vi "Time Data Filtering (V1.00).vi"(0 "wFormDSP ref in":refnum<class "GSwFormDSP.lvclass">, 5 "error in (no error)":errorcluster, 7 "Application Name":string="GenUtil", 9 "State Queue":string[](array[string])=["SC >>> Initialize"]) -> (19 "error out":errorcluster)   [LabVIEW 2022 SP3, in "SigMath.lvclass"]
uses:
  SigMath.lvclass
  API/GSwFormDSP_class/GSwFormDSP.lvclass
  <vilib>/Analysis/2dsp.llb/1D Convolution (DBL).vi
  <vilib>/Analysis/2dsp.llb/Complex FFT.vi
  W:/projects/archives/23 Charette AI Group/SPWB/API/Generic Utilities_class/Generic Utilities.lvclass
  <vilib>/Analysis/baseanly.llb/IIR Cascade Filter (DBL).vi
  API/Generic Utilities_class/Generic Utilities.lvclass
  <vilib>/Analysis/NI_AALBase.lvlib
  <vilib>/Analysis/NI_AALPro.lvlib
  <vilib>/addons/_AddQ/G#Object/G#Object.lvclass
  File IO/TDMS_class/TDMS.lvclass
panel:
  in  "GUI View":enum32{"Interface", "Admin"}(tab)
  in  "Filter Source":T1(ring)
  out "Magnitude Graph":dbl[](graph)
  out "Phase Graph":dbl[](graph)
  out "Fs":dbl
  in  "Phaseless Filter":bool=TRUE
  in  "passband ripple (dB)":dbl=0.1 caption="Passband\nRipple (dB)" format="%.2f"
  in  "stopband attenuation (dB)":dbl=60.0 caption="Stopband\nAttenuation (dB)" format="%.2f"
  in  "Order":i32=8
  in  "Type":T2(ring)=enum."Elliptic"
  in  "Upper Cut Off Freq":dbl=1000.0 format="%#.3f"
  in  "Cut Off Freq":dbl=600.0 format="%#.3f"
  in  "Filter":T3(ring)
  in  "Include Fade IN and OUT":bool
  in  "Apply":bool
  out "State History":string[](array[string])
  out "State Index":i32
  # "Filter Response"
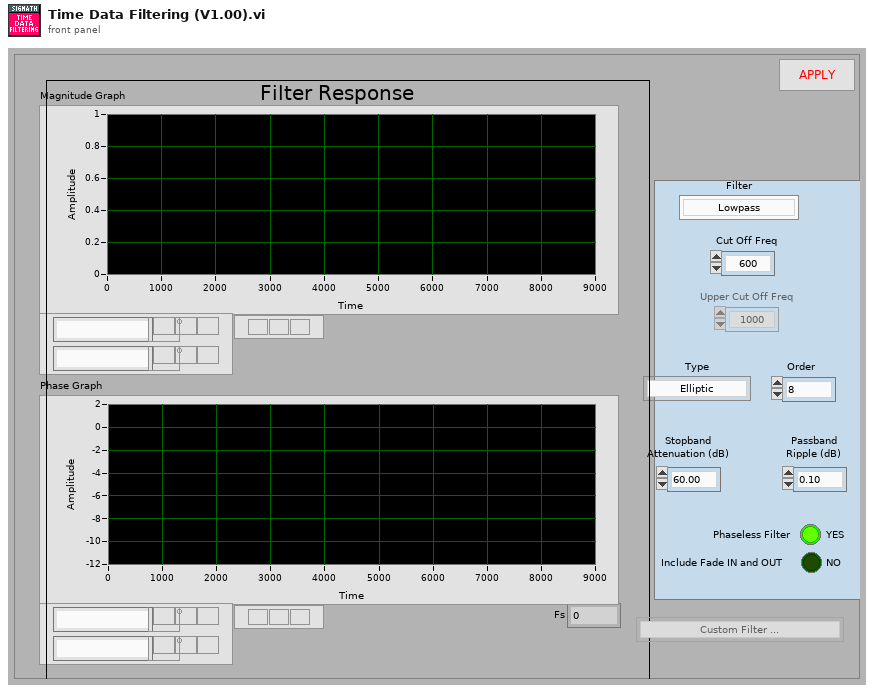
[diagram p1: front panel]
types:
  T1 = enum16{"Custom Filter ...", "Import Impulse Response (TDMS File)"}
  T2 = enum16{"Butterworth", "Chebyshev", "Inv Chebyshev", "Elliptic", "Bessel"}
  T3 = enum32{"Lowpass", "Highpass", "Bandpass", "Bandstop"}
  T4 = enum32{"Invalid", "Standard", "Closed", "Hidden", "Minimized", "Maximized"}
  T5 = enum8{"Enabled", "Disabled", "Disabled and Grayed Out"}
  T6 = typedef "SigMath.lvclass/SigMath Data.ctl" = cluster{"New Time Data Obj?":bool, "GSwFormDSP":refnum<class "GSwFormDSP.lvclass">}
  T7 = typedef "GSwFormDSP.lvclass/TDF Parameters.ctl" = cluster{"Filter":enum32{"Lowpass", "Highpass", "Bandpass", "Bandstop"}, "Type:":enum16{"Butterworth", "Chebyshev", "Inv Chebyshev", "Elliptic", "Bessel"}, "LP cutoff freq":dbl, "HP cutoff freq":dbl, "Order":i32, "passband ripple (dB)":dbl, "stopband attenuation (dB)":dbl, "Phaseless Filter":bool, "Include Fade IN and OUT":bool}
  T8 = cluster{"filter structure":enum32{"IIR 2nd Order", "IIR 4th Order"}, "Reverse Coefficients":dbl[], "Forward Coefficients":dbl[]}
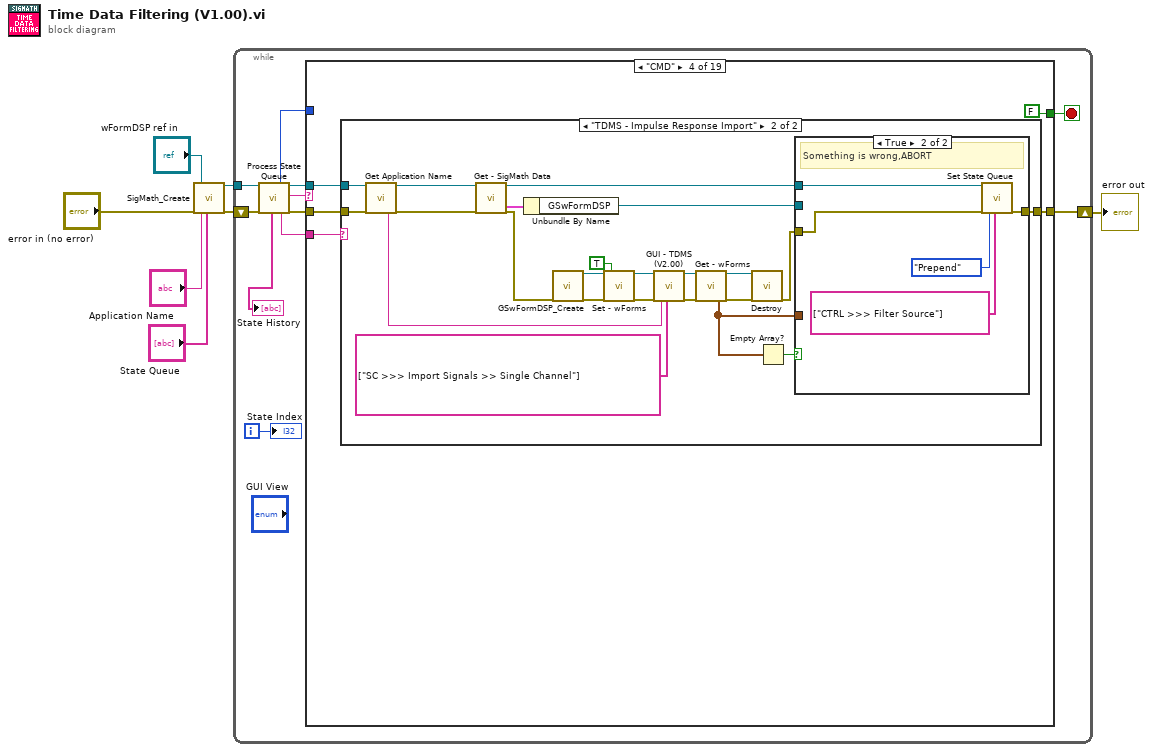
[diagram p0: block diagram]
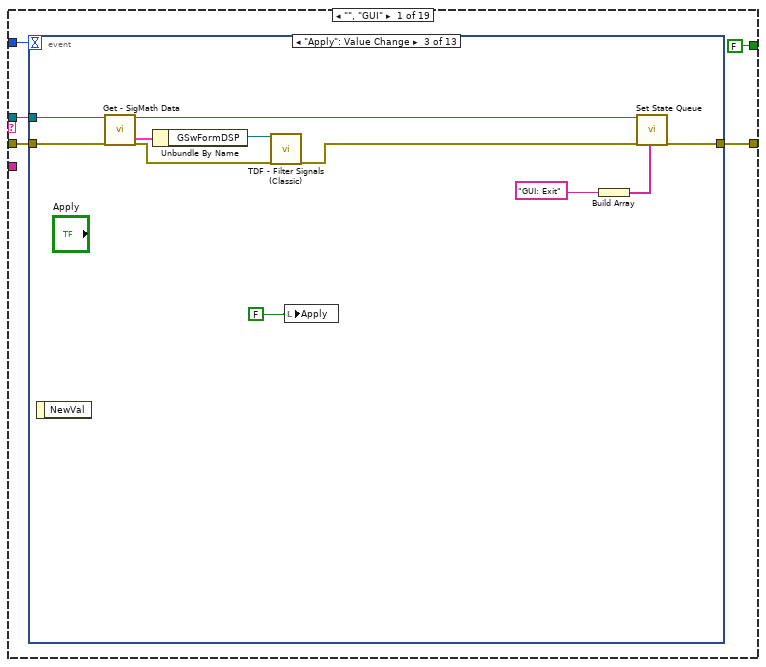
[diagram p2: hidden frame]
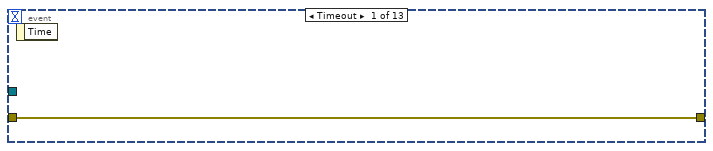
[diagram p3: hidden frame]
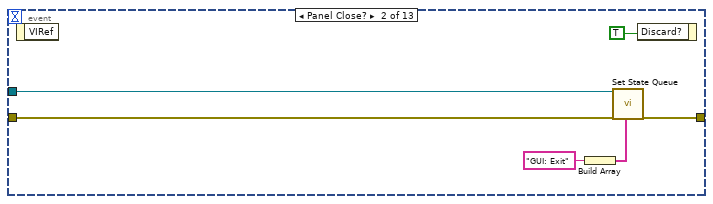
[diagram p4: hidden frame]
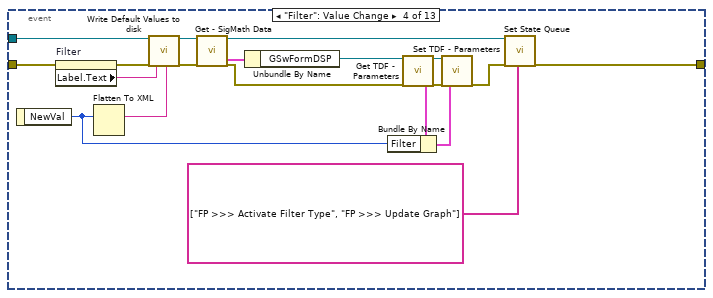
[diagram p5: hidden frame]
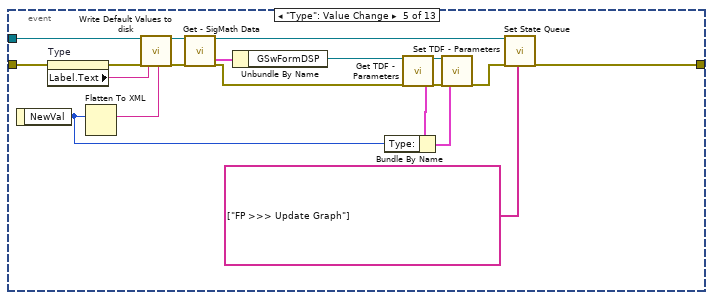
[diagram p6: hidden frame]
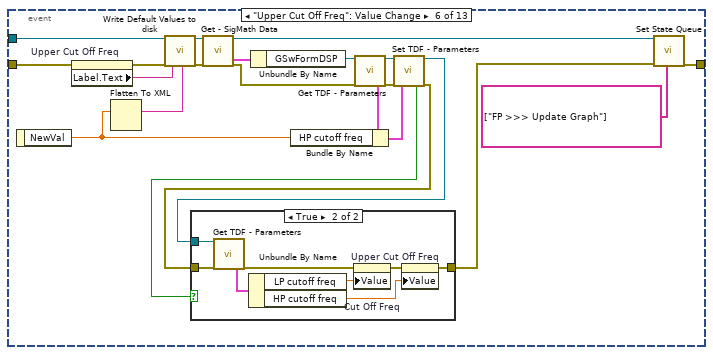
[diagram p7: hidden frame]
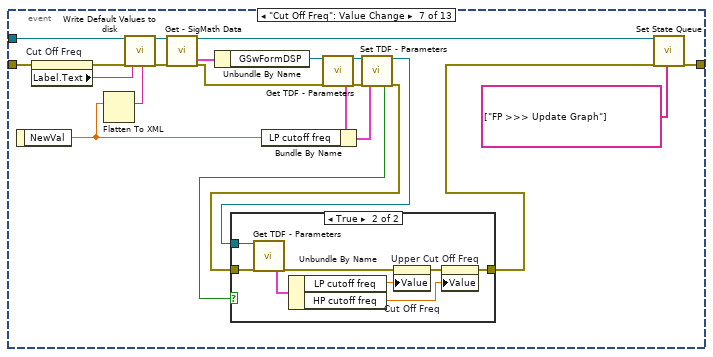
[diagram p9: hidden frame]
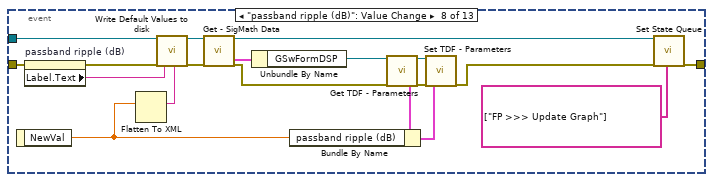
[diagram p11: hidden frame]
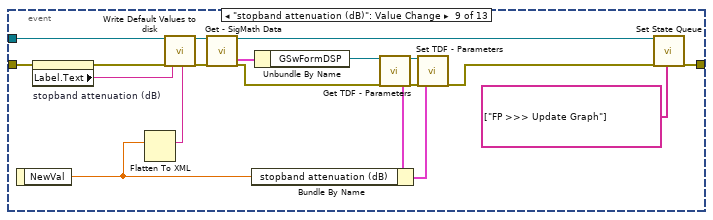
[diagram p12: hidden frame]
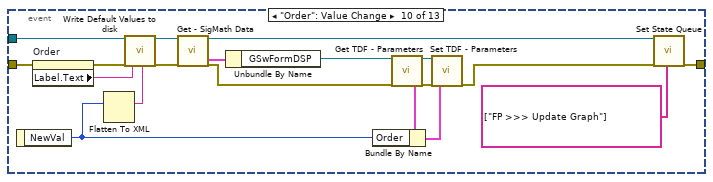
[diagram p13: hidden frame]
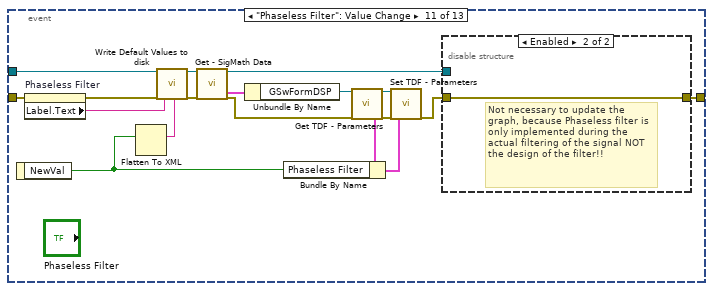
[diagram p14: hidden frame]
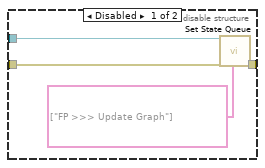
[diagram p15: hidden frame]
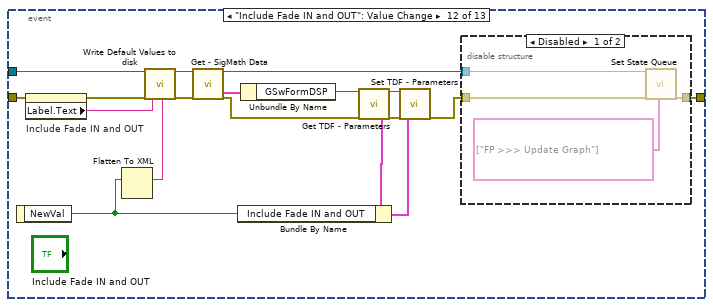
[diagram p16: hidden frame]
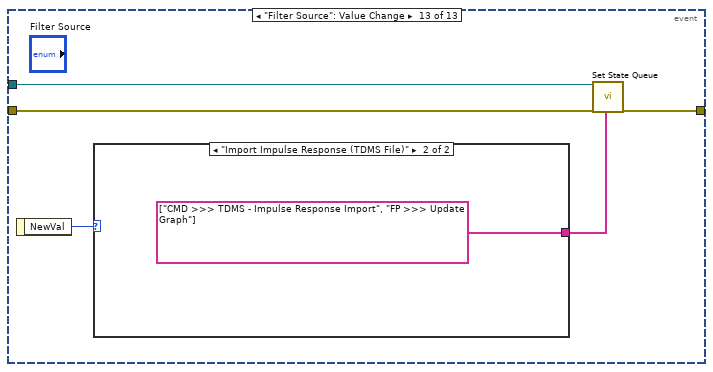
[diagram p18: hidden frame]
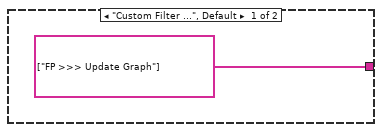
[diagram p19: hidden frame]
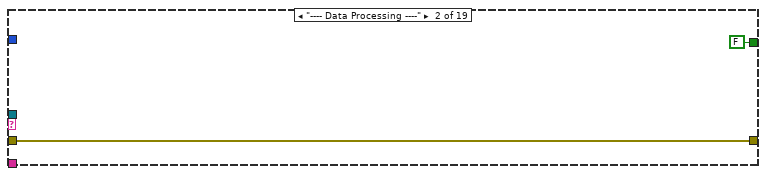
[diagram p20: hidden frame]
diagram:
  n1 = call "SigMath_Create.vi"("error in (no error)"="error in (no error)", "Time Data"="wFormDSP ref in", "Application Name"="Application Name", "State Queue"="State Queue") -> ("reference out"=w7:refnum<class "SigMath.lvclass">, "error out"=w6:errorcluster)  [unwired: 14 in]
  n2 = while {
    shift-right: [w10] -> w2
    shift-left: w6 -> [w15]
    tunnel: w7 -> [w16]
    i -> [w17]
    stop <- w18 stop-if-true
    n3 = call "Process State Queue.vi"("reference in"=w16, "error in (no error)"=w15) -> ("State History"=→"State History":string[], "Timeout"=w14:i32, "State Option"=w9:string, "reference out"=w13:refnum<class "SigMath.lvclass">, "Current State"=w12:string, "error out"=w11:errorcluster)  [unwired: 10 in, 2 out]
    n4 = case shown="\"CMD\"" w12 {
      selector: w12 -> [_ _ _ _ _ _ _ _ _ _ _ _ _ _ _ w812 _ _ _]
      tunnel: w13 -> [w21 _ _ w256 _ w306 _ w319 w609 _ w720 w733 w769 w794 _ _ _ _ w822]
      tunnel: [FALSE FALSE FALSE FALSE FALSE FALSE FALSE FALSE FALSE FALSE FALSE TRUE FALSE FALSE FALSE FALSE FALSE FALSE TRUE] -> w18
      tunnel: w14 -> [w22 _ _ _ _ _ _ _ _ _ _ _ _ _ _ _ _ _ _]
      tunnel: w9 -> [_ _ _ w259 _ w302 _ w320 w606 _ _ _ w778 _ _ _ _ _ _]
      tunnel: w11 -> [w20 w252 w254 w257 w299 w305 w315 w317 w608 w711 w716 w730 w768 w795 w808 w810 w815 w818 w821]
      tunnel: [w19 w252 w254 w258 w299 w304 w315 w318 w607 w711 w717 w729 w766 w791 w808 w810 errorcluster {"status"=FALSE, "code"=0, "source"=""} ("error out") w818 w820] -> w10
      frame "", "GUI" {
        n5 = event shown="[2] \"Apply\": Value Change" {
          selector: _ -> [_ _ _ _ _ _ _ _ _ _ _ _ _]
          dyn-events: _ -> [_ _ _ _ _ _ _ _ _ _ _ _ _]
          timeout: w22 -> [_ _ _ _ _ _ _ _ _ _ _ _ _]
          tunnel: w21 -> [_ w28 w36 w60 w79 w92 w123 w150 w169 w188 w207 w230 w246]
          tunnel: w20 -> [w24 w27 w35 w57 w76 w91 w122 w149 w168 w187 w206 w229 w247]
          tunnel: [w24 w26 w40 w48 w67 w93 w124 w151 w170 w189 w208 w231 w248] -> w19
          event Timeout {
            n6 = event-data() -> ()  [unwired: 1 in, 1 out]
          }
          event Panel Close? {
            n7 = event-data() -> ()  [unwired: 1 in, 1 out]
            n8 = Build Array("GUI: Exit") -> (w25:string[])
            n9 = call "Set State Queue.vi"("reference in"=w28, "error in (no error)"=w27, "State Queue"=w25) -> ("error out"=w26:errorcluster)  [unwired: 15 in, 1 out]
            n10 = event-data("Discard?"=TRUE) -> ()  [unwired: 1 in, 1 out]
          }
          event "Apply": Value Change {
            n11 = event-data() -> ()  [unwired: 1 in, 1 out]
            n12 = call "Get - SigMath Data.vi"("reference in"=w36, "error in (no error)"=w35) -> ("SigMath Data"=w37:T6, "reference out"=w31:refnum<class "SigMath.lvclass">, "error out"=w33:errorcluster)  [unwired: 15 in]
            n13 = Unbundle By Name(w37) -> ("GSwFormDSP"=w34:refnum<class "GSwFormDSP.lvclass">)
            n14 = call "TDF - Filter Signals (Classic).vi"("reference in"=w34, "error in (no error)"=w33) -> ("error out"=w32:errorcluster)  [unwired: 16 in, 1 out]
            n15 = local write "Apply"(FALSE ("Exit")) -> ()
            n16 = Build Array("GUI: Exit") -> (w39:string[])
            n17 = call "Set State Queue.vi"("reference in"=w31, "error in (no error)"=w32, "State Queue"=w39) -> ("error out"=w40:errorcluster)  [unwired: 15 in, 1 out]
          }
          event "Filter": Value Change {
            n18 = event-data() -> ("NewVal"=w54:T3)  [unwired: 1 in]
            n19 = property on="Filter" class="Enum (strict)"(error in=w57) -> (error out=w56:errorcluster, "Label.Text"=w59:string)  [unwired: 1 in, 1 out]
            n20 = Flatten To XML(6:w54) -> (2:w58:string)
            n21 = call-dynamic "Write Default Values to disk.vi"("reference in"=w60, "error in (no error)"=w56, "Control Label"=w59, "Value (XML String)"=w58) -> ("reference out"=w46:refnum<class "SigMath.lvclass">, "error out"=w45:errorcluster)  [unwired: 14 in]
            n22 = call "Get - SigMath Data.vi"("reference in"=w46, "error in (no error)"=w45) -> ("SigMath Data"=w47:T6, "reference out"=w43:refnum<class "SigMath.lvclass">, "error out"=w42:errorcluster)  [unwired: 15 in]
            n23 = Unbundle By Name(w47) -> ("GSwFormDSP"=w44:refnum<class "GSwFormDSP.lvclass">)
            n24 = call "Get TDF - Parameters.vi"("reference in"=w44, "error in (no error)"=w42) -> ("TDF Parameters"=w55:T7, "reference out"=w53:refnum<class "GSwFormDSP.lvclass">, "error out"=w52:errorcluster)  [unwired: 15 in]
            n25 = Bundle By Name(cluster=w55, "Filter"=w54) -> (w51:T7)
            n26 = call "Set TDF - Parameters.vi"("reference in"=w53, "error in (no error)"=w52, "TDF Parameters"=w51) -> ("error out"=w50:errorcluster)  [unwired: 14 in, 2 out]
            n27 = call "Set State Queue.vi"("reference in"=w43, "error in (no error)"=w50, "State Queue"=string[] ["FP >>> Activate Filter Type", "FP >>> Update Graph"]) -> ("error out"=w48:errorcluster)  [unwired: 15 in, 1 out]
          }
          event "Type": Value Change {
            n28 = event-data() -> ("NewVal"=w73:T2)  [unwired: 1 in]
            n29 = property on="Type" class="Enum (strict)"(error in=w76) -> (error out=w75:errorcluster, "Label.Text"=w78:string)  [unwired: 1 in, 1 out]
            n30 = Flatten To XML(6:w73) -> (2:w77:string)
            n31 = call-dynamic "Write Default Values to disk.vi"("reference in"=w79, "error in (no error)"=w75, "Control Label"=w78, "Value (XML String)"=w77) -> ("reference out"=w65:refnum<class "SigMath.lvclass">, "error out"=w64:errorcluster)  [unwired: 14 in]
            n32 = call "Get - SigMath Data.vi"("reference in"=w65, "error in (no error)"=w64) -> ("SigMath Data"=w66:T6, "reference out"=w61:refnum<class "SigMath.lvclass">, "error out"=w62:errorcluster)  [unwired: 15 in]
            n33 = Unbundle By Name(w66) -> ("GSwFormDSP"=w63:refnum<class "GSwFormDSP.lvclass">)
            n34 = call "Get TDF - Parameters.vi"("reference in"=w63, "error in (no error)"=w62) -> ("TDF Parameters"=w74:T7, "reference out"=w72:refnum<class "GSwFormDSP.lvclass">, "error out"=w71:errorcluster)  [unwired: 15 in]
            n35 = Bundle By Name(cluster=w74, "Type:"=w73) -> (w70:T7)
            n36 = call "Set TDF - Parameters.vi"("reference in"=w72, "error in (no error)"=w71, "TDF Parameters"=w70) -> ("error out"=w69:errorcluster)  [unwired: 14 in, 2 out]
            n37 = call "Set State Queue.vi"("reference in"=w61, "error in (no error)"=w69, "State Queue"=string[] ["FP >>> Update Graph"]) -> ("error out"=w67:errorcluster)  [unwired: 15 in, 1 out]
          }
          event "Upper Cut Off Freq": Value Change {
            n38 = event-data() -> ("NewVal"=w90:dbl)  [unwired: 1 in]
            n39 = property on="Upper Cut Off Freq" class="DigNum (strict)"(error in=w91) -> (error out=w99:errorcluster, "Label.Text"=w101:string)  [unwired: 1 in, 1 out]
            n40 = Flatten To XML(6:w90) -> (2:w100:string)
            n41 = call-dynamic "Write Default Values to disk.vi"("reference in"=w92, "error in (no error)"=w99, "Control Label"=w101, "Value (XML String)"=w100) -> ("reference out"=w84:refnum<class "SigMath.lvclass">, "error out"=w83:errorcluster)  [unwired: 14 in]
            n42 = call "Get - SigMath Data.vi"("reference in"=w84, "error in (no error)"=w83) -> ("SigMath Data"=w85:T6, "reference out"=w80:refnum<class "SigMath.lvclass">, "error out"=w82:errorcluster)  [unwired: 15 in]
            n43 = Unbundle By Name(w85) -> ("GSwFormDSP"=w81:refnum<class "GSwFormDSP.lvclass">)
            n44 = call "Get TDF - Parameters.vi"("reference in"=w81, "error in (no error)"=w82) -> ("TDF Parameters"=w98:T7, "reference out"=w97:refnum<class "GSwFormDSP.lvclass">, "error out"=w96:errorcluster)  [unwired: 15 in]
            n45 = Bundle By Name(cluster=w98, "HP cutoff freq"=w90) -> (w95:T7)
            n46 = call "Set TDF - Parameters.vi"("reference in"=w97, "error in (no error)"=w96, "TDF Parameters"=w95) -> ("Cut Off Freq. Coerced?"=w88:bool, "reference out"=w86:refnum<class "GSwFormDSP.lvclass">, "error out"=w89:errorcluster)  [unwired: 14 in]
            n47 = case shown="True" w88 {
              tunnel: [w102 w105] -> w87
              tunnel: w89 -> [w102 w110]
              tunnel: w86 -> [_ w109]
              frame False {
              }
              frame True {
                n48 = call "Get TDF - Parameters.vi"("reference in"=w109, "error in (no error)"=w110) -> ("TDF Parameters"=w108:T7, "error out"=w106:errorcluster)  [unwired: 15 in, 1 out]
                n49 = Unbundle By Name(w108) -> ("LP cutoff freq"=w107:dbl, "HP cutoff freq"=w103:dbl)
                n50 = property on="Cut Off Freq" class="DigNum (strict)"(error in=w106, "Value"=w107) -> (error out=w104:errorcluster)  [unwired: 1 in, 1 out]
                n51 = property on="Upper Cut Off Freq" class="DigNum (strict)"(error in=w104, "Value"=w103) -> (error out=w105:errorcluster)  [unwired: 1 in, 1 out]
              }
            }
            n52 = call "Set State Queue.vi"("reference in"=w80, "error in (no error)"=w87, "State Queue"=string[] ["FP >>> Update Graph"]) -> ("error out"=w93:errorcluster)  [unwired: 15 in, 1 out]
          }
          event "Cut Off Freq": Value Change {
            n53 = event-data() -> ("NewVal"=w121:dbl)  [unwired: 1 in]
            n54 = property on="Cut Off Freq" class="DigNum (strict)"(error in=w122) -> (error out=w130:errorcluster, "Label.Text"=w132:string)  [unwired: 1 in, 1 out]
            n55 = Flatten To XML(6:w121) -> (2:w131:string)
            n56 = call-dynamic "Write Default Values to disk.vi"("reference in"=w123, "error in (no error)"=w130, "Control Label"=w132, "Value (XML String)"=w131) -> ("reference out"=w115:refnum<class "SigMath.lvclass">, "error out"=w114:errorcluster)  [unwired: 14 in]
            n57 = call "Get - SigMath Data.vi"("reference in"=w115, "error in (no error)"=w114) -> ("SigMath Data"=w116:T6, "reference out"=w111:refnum<class "SigMath.lvclass">, "error out"=w112:errorcluster)  [unwired: 15 in]
            n58 = Unbundle By Name(w116) -> ("GSwFormDSP"=w113:refnum<class "GSwFormDSP.lvclass">)
            n59 = call "Get TDF - Parameters.vi"("reference in"=w113, "error in (no error)"=w112) -> ("TDF Parameters"=w129:T7, "reference out"=w128:refnum<class "GSwFormDSP.lvclass">, "error out"=w127:errorcluster)  [unwired: 15 in]
            n60 = Bundle By Name(cluster=w129, "LP cutoff freq"=w121) -> (w126:T7)
            n61 = call "Set TDF - Parameters.vi"("reference in"=w128, "error in (no error)"=w127, "TDF Parameters"=w126) -> ("Cut Off Freq. Coerced?"=w117:bool, "reference out"=w120:refnum<class "GSwFormDSP.lvclass">, "error out"=w119:errorcluster)  [unwired: 14 in]
            n62 = case shown="True" w117 {
              tunnel: [w133 w136] -> w118
              tunnel: w119 -> [w133 w141]
              tunnel: w120 -> [_ w140]
              frame False {
              }
              frame True {
                n63 = call "Get TDF - Parameters.vi"("reference in"=w140, "error in (no error)"=w141) -> ("TDF Parameters"=w139:T7, "error out"=w137:errorcluster)  [unwired: 15 in, 1 out]
                n64 = Unbundle By Name(w139) -> ("LP cutoff freq"=w138:dbl, "HP cutoff freq"=w134:dbl)
                n65 = property on="Cut Off Freq" class="DigNum (strict)"(error in=w137, "Value"=w138) -> (error out=w135:errorcluster)  [unwired: 1 in, 1 out]
                n66 = property on="Upper Cut Off Freq" class="DigNum (strict)"(error in=w135, "Value"=w134) -> (error out=w136:errorcluster)  [unwired: 1 in, 1 out]
              }
            }
            n67 = call "Set State Queue.vi"("reference in"=w111, "error in (no error)"=w118, "State Queue"=string[] ["FP >>> Update Graph"]) -> ("error out"=w124:errorcluster)  [unwired: 15 in, 1 out]
          }
          event "passband ripple (dB)": Value Change {
            n68 = event-data() -> ("NewVal"=w148:dbl)  [unwired: 1 in]
            n69 = property on="passband ripple (dB)" class="DigNum (strict)"(error in=w149) -> (error out=w158:errorcluster, "Label.Text"=w160:string)  [unwired: 1 in, 1 out]
            n70 = Flatten To XML(6:w148) -> (2:w159:string)
            n71 = call-dynamic "Write Default Values to disk.vi"("reference in"=w150, "error in (no error)"=w158, "Control Label"=w160, "Value (XML String)"=w159) -> ("reference out"=w146:refnum<class "SigMath.lvclass">, "error out"=w145:errorcluster)  [unwired: 14 in]
            n72 = call "Get - SigMath Data.vi"("reference in"=w146, "error in (no error)"=w145) -> ("SigMath Data"=w147:T6, "reference out"=w142:refnum<class "SigMath.lvclass">, "error out"=w143:errorcluster)  [unwired: 15 in]
            n73 = Unbundle By Name(w147) -> ("GSwFormDSP"=w144:refnum<class "GSwFormDSP.lvclass">)
            n74 = call "Get TDF - Parameters.vi"("reference in"=w144, "error in (no error)"=w143) -> ("TDF Parameters"=w157:T7, "reference out"=w156:refnum<class "GSwFormDSP.lvclass">, "error out"=w155:errorcluster)  [unwired: 15 in]
            n75 = Bundle By Name(cluster=w157, "passband ripple (dB)"=w148) -> (w154:T7)
            n76 = call "Set TDF - Parameters.vi"("reference in"=w156, "error in (no error)"=w155, "TDF Parameters"=w154) -> ("error out"=w153:errorcluster)  [unwired: 14 in, 2 out]
            n77 = call "Set State Queue.vi"("reference in"=w142, "error in (no error)"=w153, "State Queue"=string[] ["FP >>> Update Graph"]) -> ("error out"=w151:errorcluster)  [unwired: 15 in, 1 out]
          }
          event "stopband attenuation (dB)": Value Change {
            n78 = event-data() -> ("NewVal"=w167:dbl)  [unwired: 1 in]
            n79 = property on="stopband attenuation (dB)" class="DigNum (strict)"(error in=w168) -> (error out=w177:errorcluster, "Label.Text"=w179:string)  [unwired: 1 in, 1 out]
            n80 = Flatten To XML(6:w167) -> (2:w178:string)
            n81 = call-dynamic "Write Default Values to disk.vi"("reference in"=w169, "error in (no error)"=w177, "Control Label"=w179, "Value (XML String)"=w178) -> ("reference out"=w165:refnum<class "SigMath.lvclass">, "error out"=w164:errorcluster)  [unwired: 14 in]
            n82 = call "Get - SigMath Data.vi"("reference in"=w165, "error in (no error)"=w164) -> ("SigMath Data"=w166:T6, "reference out"=w162:refnum<class "SigMath.lvclass">, "error out"=w161:errorcluster)  [unwired: 15 in]
            n83 = Unbundle By Name(w166) -> ("GSwFormDSP"=w163:refnum<class "GSwFormDSP.lvclass">)
            n84 = call "Get TDF - Parameters.vi"("reference in"=w163, "error in (no error)"=w161) -> ("TDF Parameters"=w176:T7, "reference out"=w175:refnum<class "GSwFormDSP.lvclass">, "error out"=w174:errorcluster)  [unwired: 15 in]
            n85 = Bundle By Name(cluster=w176, "stopband attenuation (dB)"=w167) -> (w173:T7)
            n86 = call "Set TDF - Parameters.vi"("reference in"=w175, "error in (no error)"=w174, "TDF Parameters"=w173) -> ("error out"=w172:errorcluster)  [unwired: 14 in, 2 out]
            n87 = call "Set State Queue.vi"("reference in"=w162, "error in (no error)"=w172, "State Queue"=string[] ["FP >>> Update Graph"]) -> ("error out"=w170:errorcluster)  [unwired: 15 in, 1 out]
          }
          event "Order": Value Change {
            n88 = event-data() -> ("NewVal"=w186:i32)  [unwired: 1 in]
            n89 = property on="Order" class="DigNum (strict)"(error in=w187) -> (error out=w196:errorcluster, "Label.Text"=w198:string)  [unwired: 1 in, 1 out]
            n90 = Flatten To XML(6:w186) -> (2:w197:string)
            n91 = call-dynamic "Write Default Values to disk.vi"("reference in"=w188, "error in (no error)"=w196, "Control Label"=w198, "Value (XML String)"=w197) -> ("reference out"=w184:refnum<class "SigMath.lvclass">, "error out"=w183:errorcluster)  [unwired: 14 in]
            n92 = call "Get - SigMath Data.vi"("reference in"=w184, "error in (no error)"=w183) -> ("SigMath Data"=w185:T6, "reference out"=w180:refnum<class "SigMath.lvclass">, "error out"=w181:errorcluster)  [unwired: 15 in]
            n93 = Unbundle By Name(w185) -> ("GSwFormDSP"=w182:refnum<class "GSwFormDSP.lvclass">)
            n94 = call "Get TDF - Parameters.vi"("reference in"=w182, "error in (no error)"=w181) -> ("TDF Parameters"=w195:T7, "reference out"=w194:refnum<class "GSwFormDSP.lvclass">, "error out"=w193:errorcluster)  [unwired: 15 in]
            n95 = Bundle By Name(cluster=w195, "Order"=w186) -> (w192:T7)
            n96 = call "Set TDF - Parameters.vi"("reference in"=w194, "error in (no error)"=w193, "TDF Parameters"=w192) -> ("error out"=w191:errorcluster)  [unwired: 14 in, 2 out]
            n97 = call "Set State Queue.vi"("reference in"=w180, "error in (no error)"=w191, "State Queue"=string[] ["FP >>> Update Graph"]) -> ("error out"=w189:errorcluster)  [unwired: 15 in, 1 out]
          }
          event "Phaseless Filter": Value Change {
            n98 = event-data() -> ("NewVal"=w205:bool)  [unwired: 1 in]
            n99 = property on="Phaseless Filter" class="Bool (strict)"(error in=w206) -> (error out=w214:errorcluster, "Label.Text"=w216:string)  [unwired: 1 in, 1 out]
            n100 = Flatten To XML(6:w205) -> (2:w215:string)
            n101 = call-dynamic "Write Default Values to disk.vi"("reference in"=w207, "error in (no error)"=w214, "Control Label"=w216, "Value (XML String)"=w215) -> ("reference out"=w203:refnum<class "SigMath.lvclass">, "error out"=w202:errorcluster)  [unwired: 14 in]
            n102 = call "Get - SigMath Data.vi"("reference in"=w203, "error in (no error)"=w202) -> ("SigMath Data"=w204:T6, "reference out"=w199:refnum<class "SigMath.lvclass">, "error out"=w200:errorcluster)  [unwired: 15 in]
            n103 = Unbundle By Name(w204) -> ("GSwFormDSP"=w201:refnum<class "GSwFormDSP.lvclass">)
            n104 = call "Get TDF - Parameters.vi"("reference in"=w201, "error in (no error)"=w200) -> ("TDF Parameters"=w213:T7, "reference out"=w212:refnum<class "GSwFormDSP.lvclass">, "error out"=w211:errorcluster)  [unwired: 15 in]
            n105 = Bundle By Name(cluster=w213, "Phaseless Filter"=w205) -> (w210:T7)
            n106 = call "Set TDF - Parameters.vi"("reference in"=w212, "error in (no error)"=w211, "TDF Parameters"=w210) -> ("error out"=w209:errorcluster)  [unwired: 14 in, 2 out]
            n107 = disable-structure shown="Enabled" {
              disable-tunnel: w199 -> [w220 _]
              disable-tunnel: w209 -> [w219 w221]
              disable-tunnel: [w217 w221] -> w208
              frame Disabled {
                n108 = call "Set State Queue.vi"("reference in"=w220, "error in (no error)"=w219, "State Queue"=string[] ["FP >>> Update Graph"]) -> ("error out"=w217:errorcluster)  [unwired: 15 in, 1 out]
              }
              frame Enabled {
                # "Not necessary to update the graph, because Phaseless filter is only implemented during the actual filtering of the signal NOT the design of the filter!!"
              }
            }
          }
          event "Include Fade IN and OUT": Value Change {
            n109 = event-data() -> ("NewVal"=w228:bool)  [unwired: 1 in]
            n110 = property on="Include Fade IN and OUT" class="Bool (strict)"(error in=w229) -> (error out=w237:errorcluster, "Label.Text"=w239:string)  [unwired: 1 in, 1 out]
            n111 = Flatten To XML(6:w228) -> (2:w238:string)
            n112 = call-dynamic "Write Default Values to disk.vi"("reference in"=w230, "error in (no error)"=w237, "Control Label"=w239, "Value (XML String)"=w238) -> ("reference out"=w223:refnum<class "SigMath.lvclass">, "error out"=w226:errorcluster)  [unwired: 14 in]
            n113 = call "Get - SigMath Data.vi"("reference in"=w223, "error in (no error)"=w226) -> ("SigMath Data"=w227:T6, "reference out"=w222:refnum<class "SigMath.lvclass">, "error out"=w224:errorcluster)  [unwired: 15 in]
            n114 = Unbundle By Name(w227) -> ("GSwFormDSP"=w225:refnum<class "GSwFormDSP.lvclass">)
            n115 = call "Get TDF - Parameters.vi"("reference in"=w225, "error in (no error)"=w224) -> ("TDF Parameters"=w236:T7, "reference out"=w235:refnum<class "GSwFormDSP.lvclass">, "error out"=w234:errorcluster)  [unwired: 15 in]
            n116 = Bundle By Name(cluster=w236, "Include Fade IN and OUT"=w228) -> (w233:T7)
            n117 = call "Set TDF - Parameters.vi"("reference in"=w235, "error in (no error)"=w234, "TDF Parameters"=w233) -> ("error out"=w232:errorcluster)  [unwired: 14 in, 2 out]
            n118 = disable-structure shown="Disabled" {
              disable-tunnel: w232 -> [w243 w244]
              disable-tunnel: [w241 w244] -> w231
              disable-tunnel: w222 -> [w240 _]
              frame Disabled {
                n119 = call "Set State Queue.vi"("reference in"=w240, "error in (no error)"=w243, "State Queue"=string[] ["FP >>> Update Graph"]) -> ("error out"=w241:errorcluster)  [unwired: 15 in, 1 out]
              }
              frame Enabled {
                # "Not necessary to update the graph, because Phase IN/OUT is only valid during the actual filtering of the signal NOT the design of the filter!!"
              }
            }
          }
          event "Filter Source": Value Change {
            n120 = event-data() -> ("NewVal"=w245:T1)  [unwired: 1 in]
            n121 = case shown="\"Import Impulse Response (TDMS File)\"" w245 {
              tunnel: [string[] ["FP >>> Update Graph"] ("State Queue") string[] ["CMD >>> TDMS - Impulse Response Import", "FP >>> Update Graph"] ("State Queue")] -> w249
              frame "Custom Filter ...", Default {
              }
              frame "Import Impulse Response (TDMS File)" {
              }
            }
            n122 = call "Set State Queue.vi"("reference in"=w246, "error in (no error)"=w247, "State Queue"=w249) -> ("error out"=w248:errorcluster)  [unwired: 15 in, 1 out]
          }
        }
      }
      frame "---- Data Processing ----" {
      }
      frame "---- Command ----" {
      }
      frame "CMD" {
        n123 = case shown="\"TDMS - Impulse Response Import\"" w259 {
          selector: w259 -> [w262 _]
          tunnel: [w261 w266] -> w258
          tunnel: w257 -> [w261 w286]
          tunnel: w256 -> [_ w285]
          frame "", Default {
            n124 = Concatenate Strings("The following \"CMD\" is unrecognized:\n", w262) -> (w263:string)
            n125 = One Button Dialog(message=w263) -> ()  [unwired: 1 in, 1 out]
          }
          frame "TDMS - Impulse Response Import" {
            n126 = call "Get Application Name.vi"("reference in"=w285, "error in (no error)"=w286) -> ("Application Name"=w279:string, "reference out"=w273:refnum<class "SigMath.lvclass">, "error out"=w272:errorcluster)  [unwired: 15 in]
            n127 = call "Get - SigMath Data.vi"("reference in"=w273, "error in (no error)"=w272) -> ("SigMath Data"=w274:T6, "reference out"=w265:refnum<class "SigMath.lvclass">, "error out"=w271:errorcluster)  [unwired: 15 in]
            n128 = Unbundle By Name(w274) -> ("GSwFormDSP"=w269:refnum<class "GSwFormDSP.lvclass">)
            n129 = call "GSwFormDSP_Create.vi"("error in (no error)"=w271) -> ("reference out"=w283:refnum<class "GSwFormDSP.lvclass">, "error out"=w281:errorcluster)  [unwired: 17 in]
            n130 = call "Set - wForms.vi"("reference in"=w283, "error in (no error)"=w281, "Init wForms"=TRUE) -> ("reference out"=w282:refnum<class "GSwFormDSP.lvclass">, "error out"=w280:errorcluster)  [unwired: 15 in]
            n131 = call "GUI - TDMS (V2.00).vi"("Time Data IN"=w282, "error in (no error)"=w280, "Application Name"=w279, "State Queue"=string[] ["SC >>> Import Signals >> Single Channel"]) -> ("SubVI Time Data DUP"=w277:refnum<class "GSwFormDSP.lvclass">, "error out"=w278:errorcluster)  [unwired: 13 in, 1 out]
            n132 = call-dynamic "Get - wForms.vi"("reference in"=w277, "error in (no error)"=w278) -> ("wForms"=w268:waveform(dbl)[], "reference out"=w275:refnum<class "GSwFormDSP.lvclass">, "error out"=w276:errorcluster)  [unwired: 14 in, 1 out]
            n133 = call-dynamic "Destroy.vi"("reference in"=w275, "error in (no error)"=w276) -> ("error out"=w267:errorcluster)  [unwired: 16 in, 1 out]
            n134 = Empty Array?(array=w268) -> (empty?=w270:bool)
            n135 = case shown="True" w270 {
              tunnel: w269 -> [w293 _]
              tunnel: w268 -> [w291 _]
              tunnel: w267 -> [w290 w295]
              tunnel: [w288 w294] -> w266
              tunnel: w265 -> [_ w298]
              frame False {
                # "Filter loaded, continue"
                n136 = Index Array(array=w291, index=0) -> (element=w289:waveform(dbl))
                n137 = call "Set TDF - Filter Impulse response.vi"("reference in"=w293, "error in (no error)"=w290, "Filter Impulse Response (TDF)"=w289) -> ("error out"=w288:errorcluster)  [unwired: 15 in, 1 out]
              }
              frame True {
                # "Something is wrong,ABORT"
                n138 = call "Set State Queue.vi"("reference in"=w298, "error in (no error)"=w295, "State Queue Options"=enum16{"Replace", "Append", "Prepend"}."Prepend", "State Queue"=string[] ["CTRL >>> Filter Source"]) -> ("error out"=w294:errorcluster)  [unwired: 14 in, 1 out]
              }
            }
          }
        }
      }
      frame "---- Scripts ----" {
      }
      frame "SC" {
        n139 = case shown="\"Initialize\"" w302 {
          selector: w302 -> [w310 _]
          tunnel: [string[] [] ("State Queue OUT") string[] ["GUI: Initialize Ref", "CTRL >>> Fs", "CTRL >>> Filter Source", "CTRL >>> Filter", "CTRL >>> Type", "CTRL >>> Low Cut Off Freq", "CTRL >>> Upper Cut Off Freq", "CTRL >>> Pass Band Ripple", "CTRL >>> Stop Band Attenuation", "CTRL >>> Phaseless Filter", "CTRL >>> Fade In and OUT", "CTRL >>> Filter Order", "FP >>> Activate Filter Type", "FP >>> Open", "FP >>> Update Graph"] ("State Queue OUT")] -> w303
          tunnel: [enum16{"Replace", "Append", "Prepend"}."Append" ("State Queue Options") enum16{"Replace", "Append", "Prepend"}."Append" ("State Queue Options")] -> w301
          frame "False", Default {
            n140 = Concatenate Strings("The following \"Script\" is unrecognized:\n", w310) -> (w311:string)
            n141 = One Button Dialog(message=w311) -> ()  [unwired: 1 in, 1 out]
          }
          frame "Initialize" {
          }
        }
        n142 = call "Set State Queue.vi"("reference in"=w306, "error in (no error)"=w305, "State Queue Options"=w301, "State Queue"=w303) -> ("error out"=w304:errorcluster)  [unwired: 14 in, 1 out]
      }
      frame "---- Front Panel Mgmt ----" {
      }
      frame "CTRL" {
        n143 = case shown="\"Filter Source\"" w320 {
          selector: w320 -> [w324 _ _ _ _ _ _ _ _ _ _ _]
          tunnel: w319 -> [_ w342 w369 w399 w438 w474 w501 w528 w555 w582 w596 _]
          tunnel: [w322 w333 w360 w387 w426 w465 w492 w519 w546 w573 w598 w605] -> w318
          tunnel: w317 -> [w322 w340 w367 w397 w436 w472 w499 w526 w553 w580 w595 w605]
          frame "unknown", Default {
            n144 = Concatenate Strings("The following control name is unrecognized:\n", w324) -> (w323:string)
            n145 = One Button Dialog(message=w323) -> ()  [unwired: 1 in, 1 out]
          }
          frame "Filter" {
            n146 = property on="Filter" class="Enum (strict)"(error in=w340) -> (error out=w341:errorcluster, "Label.Text"=w339:string, "Value"=w344:T3)  [unwired: 1 in, 1 out]
            n147 = call-dynamic "Read Default Values from Disk.vi"("reference in"=w342, "error in (no error)"=w341, "Control Label"=w339) -> ("Value (XML String)"=w326:string, "reference out"=w327:refnum<class "SigMath.lvclass">, "error out"=w338:errorcluster)  [unwired: 14 in]
            n148 = case shown="\"anything\", Default" w326 {
              selector: w326 -> [w350 _]
              tunnel: [w345 w352] -> w332
              tunnel: w344 -> [w347 w352]
              tunnel: w338 -> [w348 w351]
              tunnel: [w348 w351] -> w343
              frame "anything", Default {
                n149 = Unflatten From XML(xml string=w350, type=w347, error in (no error)=w348) -> (value=w346:T3, error out=w349:errorcluster)
                n150 = Select(t=w347, s=w349, f=w346) -> (s? t:f=w345:T3)
              }
              frame "" {
                # "Either the file was not found or there was some error"
              }
            }
            n151 = property on="Filter" class="Enum (strict)"(error in=w343, "Value"=w332) -> (error out=w330:errorcluster)  [unwired: 1 in, 1 out]
            n152 = call "Get - SigMath Data.vi"("reference in"=w327, "error in (no error)"=w330) -> ("SigMath Data"=w331:T6, "error out"=w328:errorcluster)  [unwired: 15 in, 1 out]
            n153 = Unbundle By Name(w331) -> ("GSwFormDSP"=w329:refnum<class "GSwFormDSP.lvclass">)
            n154 = call "Get TDF - Parameters.vi"("reference in"=w329, "error in (no error)"=w328) -> ("TDF Parameters"=w334:T7, "reference out"=w335:refnum<class "GSwFormDSP.lvclass">, "error out"=w336:errorcluster)  [unwired: 15 in]
            n155 = Bundle By Name(cluster=w334, "Filter"=w332) -> (w337:T7)
            n156 = call "Set TDF - Parameters.vi"("reference in"=w335, "error in (no error)"=w336, "TDF Parameters"=w337) -> ("error out"=w333:errorcluster)  [unwired: 14 in, 2 out]
          }
          frame "Type" {
            n157 = property on="Type" class="Enum (strict)"(error in=w367) -> (error out=w368:errorcluster, "Label.Text"=w366:string, "Value"=w371:T2)  [unwired: 1 in, 1 out]
            n158 = call-dynamic "Read Default Values from Disk.vi"("reference in"=w369, "error in (no error)"=w368, "Control Label"=w366) -> ("Value (XML String)"=w353:string, "reference out"=w356:refnum<class "SigMath.lvclass">, "error out"=w365:errorcluster)  [unwired: 14 in]
            n159 = case shown="\"anything\", Default" w353 {
              selector: w353 -> [w377 _]
              tunnel: [w372 w379] -> w359
              tunnel: w371 -> [w374 w379]
              tunnel: w365 -> [w375 w378]
              tunnel: [w375 w378] -> w370
              frame "anything", Default {
                n160 = Unflatten From XML(xml string=w377, type=w374, error in (no error)=w375) -> (value=w373:T2, error out=w376:errorcluster)
                n161 = Select(t=w374, s=w376, f=w373) -> (s? t:f=w372:T2)
              }
              frame "" {
                # "Either the file was not found or there was some error"
              }
            }
            n162 = property on="Type" class="Enum (strict)"(error in=w370, "Value"=w359) -> (error out=w357:errorcluster)  [unwired: 1 in, 1 out]
            n163 = call "Get - SigMath Data.vi"("reference in"=w356, "error in (no error)"=w357) -> ("SigMath Data"=w358:T6, "error out"=w354:errorcluster)  [unwired: 15 in, 1 out]
            n164 = Unbundle By Name(w358) -> ("GSwFormDSP"=w355:refnum<class "GSwFormDSP.lvclass">)
            n165 = call "Get TDF - Parameters.vi"("reference in"=w355, "error in (no error)"=w354) -> ("TDF Parameters"=w361:T7, "reference out"=w362:refnum<class "GSwFormDSP.lvclass">, "error out"=w363:errorcluster)  [unwired: 15 in]
            n166 = Bundle By Name(cluster=w361, "Type:"=w359) -> (w364:T7)
            n167 = call "Set TDF - Parameters.vi"("reference in"=w362, "error in (no error)"=w363, "TDF Parameters"=w364) -> ("error out"=w360:errorcluster)  [unwired: 14 in, 2 out]
          }
          frame "Low Cut Off Freq" {
            n168 = property on="Cut Off Freq" class="DigNum (strict)"(error in=w397) -> (error out=w398:errorcluster, "Label.Text"=w396:string, "Value"=w401:dbl)  [unwired: 1 in, 1 out]
            n169 = call-dynamic "Read Default Values from Disk.vi"("reference in"=w399, "error in (no error)"=w398, "Control Label"=w396) -> ("Value (XML String)"=w380:string, "reference out"=w382:refnum<class "SigMath.lvclass">, "error out"=w395:errorcluster)  [unwired: 14 in]
            n170 = case shown="\"anything\", Default" w380 {
              selector: w380 -> [w416 _]
              tunnel: [w411 w418] -> w390
              tunnel: w401 -> [w413 w418]
              tunnel: w395 -> [w414 w417]
              tunnel: [w414 w417] -> w400
              frame "anything", Default {
                n171 = Unflatten From XML(xml string=w416, type=w413, error in (no error)=w414) -> (value=w412:dbl, error out=w415:errorcluster)
                n172 = Select(t=w413, s=w415, f=w412) -> (s? t:f=w411:dbl)
              }
              frame "" {
                # "Either the file was not found or there was some error"
              }
            }
            n173 = property on="Cut Off Freq" class="DigNum (strict)"(error in=w400, "Value"=w390) -> (error out=w384:errorcluster)  [unwired: 1 in, 1 out]
            n174 = call "Get - SigMath Data.vi"("reference in"=w382, "error in (no error)"=w384) -> ("SigMath Data"=w385:T6, "error out"=w381:errorcluster)  [unwired: 15 in, 1 out]
            n175 = Unbundle By Name(w385) -> ("GSwFormDSP"=w383:refnum<class "GSwFormDSP.lvclass">)
            n176 = call "Get TDF - Parameters.vi"("reference in"=w383, "error in (no error)"=w381) -> ("TDF Parameters"=w391:T7, "reference out"=w392:refnum<class "GSwFormDSP.lvclass">, "error out"=w393:errorcluster)  [unwired: 15 in]
            n177 = Bundle By Name(cluster=w391, "LP cutoff freq"=w390) -> (w394:T7)
            n178 = call "Set TDF - Parameters.vi"("reference in"=w392, "error in (no error)"=w393, "TDF Parameters"=w394) -> ("Cut Off Freq. Coerced?"=w389:bool, "reference out"=w386:refnum<class "GSwFormDSP.lvclass">, "error out"=w388:errorcluster)  [unwired: 14 in]
            n179 = case shown="True" w389 {
              tunnel: [w402 w405] -> w387
              tunnel: w388 -> [w402 w410]
              tunnel: w386 -> [_ w409]
              frame False {
              }
              frame True {
                n180 = call "Get TDF - Parameters.vi"("reference in"=w409, "error in (no error)"=w410) -> ("TDF Parameters"=w408:T7, "error out"=w406:errorcluster)  [unwired: 15 in, 1 out]
                n181 = Unbundle By Name(w408) -> ("LP cutoff freq"=w407:dbl, "HP cutoff freq"=w403:dbl)
                n182 = property on="Cut Off Freq" class="DigNum (strict)"(error in=w406, "Value"=w407) -> (error out=w404:errorcluster)  [unwired: 1 in, 1 out]
                n183 = property on="Upper Cut Off Freq" class="DigNum (strict)"(error in=w404, "Value"=w403) -> (error out=w405:errorcluster)  [unwired: 1 in, 1 out]
              }
            }
          }
          frame "Upper Cut Off Freq" {
            n184 = property on="Upper Cut Off Freq" class="DigNum (strict)"(error in=w436) -> (error out=w437:errorcluster, "Label.Text"=w435:string, "Value"=w440:dbl)  [unwired: 1 in, 1 out]
            n185 = call-dynamic "Read Default Values from Disk.vi"("reference in"=w438, "error in (no error)"=w437, "Control Label"=w435) -> ("Value (XML String)"=w419:string, "reference out"=w423:refnum<class "SigMath.lvclass">, "error out"=w434:errorcluster)  [unwired: 14 in]
            n186 = case shown="\"anything\", Default" w419 {
              selector: w419 -> [w455 _]
              tunnel: [w450 w457] -> w429
              tunnel: w440 -> [w452 w457]
              tunnel: w434 -> [w453 w456]
              tunnel: [w453 w456] -> w439
              frame "anything", Default {
                n187 = Unflatten From XML(xml string=w455, type=w452, error in (no error)=w453) -> (value=w451:dbl, error out=w454:errorcluster)
                n188 = Select(t=w452, s=w454, f=w451) -> (s? t:f=w450:dbl)
              }
              frame "" {
                # "Either the file was not found or there was some error"
              }
            }
            n189 = property on="Upper Cut Off Freq" class="DigNum (strict)"(error in=w439, "Value"=w429) -> (error out=w422:errorcluster)  [unwired: 1 in, 1 out]
            n190 = call "Get - SigMath Data.vi"("reference in"=w423, "error in (no error)"=w422) -> ("SigMath Data"=w424:T6, "error out"=w421:errorcluster)  [unwired: 15 in, 1 out]
            n191 = Unbundle By Name(w424) -> ("GSwFormDSP"=w420:refnum<class "GSwFormDSP.lvclass">)
            n192 = call "Get TDF - Parameters.vi"("reference in"=w420, "error in (no error)"=w421) -> ("TDF Parameters"=w430:T7, "reference out"=w431:refnum<class "GSwFormDSP.lvclass">, "error out"=w432:errorcluster)  [unwired: 15 in]
            n193 = Bundle By Name(cluster=w430, "HP cutoff freq"=w429) -> (w433:T7)
            n194 = call "Set TDF - Parameters.vi"("reference in"=w431, "error in (no error)"=w432, "TDF Parameters"=w433) -> ("Cut Off Freq. Coerced?"=w425:bool, "reference out"=w427:refnum<class "GSwFormDSP.lvclass">, "error out"=w428:errorcluster)  [unwired: 14 in]
            n195 = case shown="True" w425 {
              tunnel: [w441 w444] -> w426
              tunnel: w428 -> [w441 w449]
              tunnel: w427 -> [_ w448]
              frame False {
              }
              frame True {
                n196 = call "Get TDF - Parameters.vi"("reference in"=w448, "error in (no error)"=w449) -> ("TDF Parameters"=w447:T7, "error out"=w445:errorcluster)  [unwired: 15 in, 1 out]
                n197 = Unbundle By Name(w447) -> ("LP cutoff freq"=w446:dbl, "HP cutoff freq"=w442:dbl)
                n198 = property on="Cut Off Freq" class="DigNum (strict)"(error in=w445, "Value"=w446) -> (error out=w443:errorcluster)  [unwired: 1 in, 1 out]
                n199 = property on="Upper Cut Off Freq" class="DigNum (strict)"(error in=w443, "Value"=w442) -> (error out=w444:errorcluster)  [unwired: 1 in, 1 out]
              }
            }
          }
          frame "Pass Band Ripple" {
            n200 = property on="passband ripple (dB)" class="DigNum (strict)"(error in=w472) -> (error out=w473:errorcluster, "Label.Text"=w471:string, "Value"=w476:dbl)  [unwired: 1 in, 1 out]
            n201 = call-dynamic "Read Default Values from Disk.vi"("reference in"=w474, "error in (no error)"=w473, "Control Label"=w471) -> ("Value (XML String)"=w458:string, "reference out"=w462:refnum<class "SigMath.lvclass">, "error out"=w470:errorcluster)  [unwired: 14 in]
            n202 = case shown="\"anything\", Default" w458 {
              selector: w458 -> [w482 _]
              tunnel: [w477 w484] -> w464
              tunnel: w476 -> [w479 w484]
              tunnel: w470 -> [w480 w483]
              tunnel: [w480 w483] -> w475
              frame "anything", Default {
                n203 = Unflatten From XML(xml string=w482, type=w479, error in (no error)=w480) -> (value=w478:dbl, error out=w481:errorcluster)
                n204 = Select(t=w479, s=w481, f=w478) -> (s? t:f=w477:dbl)
              }
              frame "" {
                # "Either the file was not found or there was some error"
              }
            }
            n205 = property on="passband ripple (dB)" class="DigNum (strict)"(error in=w475, "Value"=w464) -> (error out=w461:errorcluster)  [unwired: 1 in, 1 out]
            n206 = call "Get - SigMath Data.vi"("reference in"=w462, "error in (no error)"=w461) -> ("SigMath Data"=w463:T6, "error out"=w460:errorcluster)  [unwired: 15 in, 1 out]
            n207 = Unbundle By Name(w463) -> ("GSwFormDSP"=w459:refnum<class "GSwFormDSP.lvclass">)
            n208 = call "Get TDF - Parameters.vi"("reference in"=w459, "error in (no error)"=w460) -> ("TDF Parameters"=w466:T7, "reference out"=w467:refnum<class "GSwFormDSP.lvclass">, "error out"=w468:errorcluster)  [unwired: 15 in]
            n209 = Bundle By Name(cluster=w466, "passband ripple (dB)"=w464) -> (w469:T7)
            n210 = call "Set TDF - Parameters.vi"("reference in"=w467, "error in (no error)"=w468, "TDF Parameters"=w469) -> ("error out"=w465:errorcluster)  [unwired: 14 in, 2 out]
          }
          frame "Stop Band Attenuation" {
            n211 = property on="stopband attenuation (dB)" class="DigNum (strict)"(error in=w499) -> (error out=w500:errorcluster, "Label.Text"=w498:string, "Value"=w503:dbl)  [unwired: 1 in, 1 out]
            n212 = call-dynamic "Read Default Values from Disk.vi"("reference in"=w501, "error in (no error)"=w500, "Control Label"=w498) -> ("Value (XML String)"=w485:string, "reference out"=w489:refnum<class "SigMath.lvclass">, "error out"=w497:errorcluster)  [unwired: 14 in]
            n213 = case shown="\"anything\", Default" w485 {
              selector: w485 -> [w509 _]
              tunnel: [w504 w511] -> w491
              tunnel: w503 -> [w506 w511]
              tunnel: w497 -> [w507 w510]
              tunnel: [w507 w510] -> w502
              frame "anything", Default {
                n214 = Unflatten From XML(xml string=w509, type=w506, error in (no error)=w507) -> (value=w505:dbl, error out=w508:errorcluster)
                n215 = Select(t=w506, s=w508, f=w505) -> (s? t:f=w504:dbl)
              }
              frame "" {
                # "Either the file was not found or there was some error"
              }
            }
            n216 = property on="stopband attenuation (dB)" class="DigNum (strict)"(error in=w502, "Value"=w491) -> (error out=w488:errorcluster)  [unwired: 1 in, 1 out]
            n217 = call "Get - SigMath Data.vi"("reference in"=w489, "error in (no error)"=w488) -> ("SigMath Data"=w490:T6, "error out"=w487:errorcluster)  [unwired: 15 in, 1 out]
            n218 = Unbundle By Name(w490) -> ("GSwFormDSP"=w486:refnum<class "GSwFormDSP.lvclass">)
            n219 = call "Get TDF - Parameters.vi"("reference in"=w486, "error in (no error)"=w487) -> ("TDF Parameters"=w493:T7, "reference out"=w494:refnum<class "GSwFormDSP.lvclass">, "error out"=w495:errorcluster)  [unwired: 15 in]
            n220 = Bundle By Name(cluster=w493, "stopband attenuation (dB)"=w491) -> (w496:T7)
            n221 = call "Set TDF - Parameters.vi"("reference in"=w494, "error in (no error)"=w495, "TDF Parameters"=w496) -> ("error out"=w492:errorcluster)  [unwired: 14 in, 2 out]
          }
          frame "Phaseless Filter" {
            n222 = property on="Phaseless Filter" class="Bool (strict)"(error in=w526) -> (error out=w527:errorcluster, "Label.Text"=w525:string, "Value"=w530:bool)  [unwired: 1 in, 1 out]
            n223 = call-dynamic "Read Default Values from Disk.vi"("reference in"=w528, "error in (no error)"=w527, "Control Label"=w525) -> ("Value (XML String)"=w512:string, "reference out"=w516:refnum<class "SigMath.lvclass">, "error out"=w524:errorcluster)  [unwired: 14 in]
            n224 = case shown="\"anything\", Default" w512 {
              selector: w512 -> [w536 _]
              tunnel: [w531 w538] -> w518
              tunnel: w530 -> [w533 w538]
              tunnel: w524 -> [w534 w537]
              tunnel: [w534 w537] -> w529
              frame "anything", Default {
                n225 = Unflatten From XML(xml string=w536, type=w533, error in (no error)=w534) -> (value=w532:bool, error out=w535:errorcluster)
                n226 = Select(t=w533, s=w535, f=w532) -> (s? t:f=w531:bool)
              }
              frame "" {
                # "Either the file was not found or there was some error"
              }
            }
            n227 = property on="Phaseless Filter" class="Bool (strict)"(error in=w529, "Value"=w518) -> (error out=w515:errorcluster)  [unwired: 1 in, 1 out]
            n228 = call "Get - SigMath Data.vi"("reference in"=w516, "error in (no error)"=w515) -> ("SigMath Data"=w517:T6, "error out"=w514:errorcluster)  [unwired: 15 in, 1 out]
            n229 = Unbundle By Name(w517) -> ("GSwFormDSP"=w513:refnum<class "GSwFormDSP.lvclass">)
            n230 = call "Get TDF - Parameters.vi"("reference in"=w513, "error in (no error)"=w514) -> ("TDF Parameters"=w520:T7, "reference out"=w521:refnum<class "GSwFormDSP.lvclass">, "error out"=w522:errorcluster)  [unwired: 15 in]
            n231 = Bundle By Name(cluster=w520, "Phaseless Filter"=w518) -> (w523:T7)
            n232 = call "Set TDF - Parameters.vi"("reference in"=w521, "error in (no error)"=w522, "TDF Parameters"=w523) -> ("error out"=w519:errorcluster)  [unwired: 14 in, 2 out]
          }
          frame "Fade In and OUT" {
            n233 = property on="Include Fade IN and OUT" class="Bool (strict)"(error in=w553) -> (error out=w554:errorcluster, "Label.Text"=w552:string, "Value"=w557:bool)  [unwired: 1 in, 1 out]
            n234 = call-dynamic "Read Default Values from Disk.vi"("reference in"=w555, "error in (no error)"=w554, "Control Label"=w552) -> ("Value (XML String)"=w539:string, "reference out"=w543:refnum<class "SigMath.lvclass">, "error out"=w551:errorcluster)  [unwired: 14 in]
            n235 = case shown="\"anything\", Default" w539 {
              selector: w539 -> [w563 _]
              tunnel: [w558 w565] -> w545
              tunnel: w557 -> [w560 w565]
              tunnel: w551 -> [w561 w564]
              tunnel: [w561 w564] -> w556
              frame "anything", Default {
                n236 = Unflatten From XML(xml string=w563, type=w560, error in (no error)=w561) -> (value=w559:bool, error out=w562:errorcluster)
                n237 = Select(t=w560, s=w562, f=w559) -> (s? t:f=w558:bool)
              }
              frame "" {
                # "Either the file was not found or there was some error"
              }
            }
            n238 = property on="Include Fade IN and OUT" class="Bool (strict)"(error in=w556, "Value"=w545) -> (error out=w542:errorcluster)  [unwired: 1 in, 1 out]
            n239 = call "Get - SigMath Data.vi"("reference in"=w543, "error in (no error)"=w542) -> ("SigMath Data"=w544:T6, "error out"=w541:errorcluster)  [unwired: 15 in, 1 out]
            n240 = Unbundle By Name(w544) -> ("GSwFormDSP"=w540:refnum<class "GSwFormDSP.lvclass">)
            n241 = call "Get TDF - Parameters.vi"("reference in"=w540, "error in (no error)"=w541) -> ("TDF Parameters"=w547:T7, "reference out"=w548:refnum<class "GSwFormDSP.lvclass">, "error out"=w549:errorcluster)  [unwired: 15 in]
            n242 = Bundle By Name(cluster=w547, "Include Fade IN and OUT"=w545) -> (w550:T7)
            n243 = call "Set TDF - Parameters.vi"("reference in"=w548, "error in (no error)"=w549, "TDF Parameters"=w550) -> ("error out"=w546:errorcluster)  [unwired: 14 in, 2 out]
          }
          frame "Filter Order" {
            n244 = property on="Order" class="DigNum (strict)"(error in=w580) -> (error out=w581:errorcluster, "Label.Text"=w579:string, "Value"=w584:i32)  [unwired: 1 in, 1 out]
            n245 = call-dynamic "Read Default Values from Disk.vi"("reference in"=w582, "error in (no error)"=w581, "Control Label"=w579) -> ("Value (XML String)"=w566:string, "reference out"=w567:refnum<class "SigMath.lvclass">, "error out"=w578:errorcluster)  [unwired: 14 in]
            n246 = case shown="\"anything\", Default" w566 {
              selector: w566 -> [w590 _]
              tunnel: [w585 w592] -> w572
              tunnel: w584 -> [w587 w592]
              tunnel: w578 -> [w588 w591]
              tunnel: [w588 w591] -> w583
              frame "anything", Default {
                n247 = Unflatten From XML(xml string=w590, type=w587, error in (no error)=w588) -> (value=w586:i32, error out=w589:errorcluster)
                n248 = Select(t=w587, s=w589, f=w586) -> (s? t:f=w585:i32)
              }
              frame "" {
                # "Either the file was not found or there was some error"
              }
            }
            n249 = property on="Order" class="DigNum (strict)"(error in=w583, "Value"=w572) -> (error out=w568:errorcluster)  [unwired: 1 in, 1 out]
            n250 = call "Get - SigMath Data.vi"("reference in"=w567, "error in (no error)"=w568) -> ("SigMath Data"=w571:T6, "error out"=w569:errorcluster)  [unwired: 15 in, 1 out]
            n251 = Unbundle By Name(w571) -> ("GSwFormDSP"=w570:refnum<class "GSwFormDSP.lvclass">)
            n252 = call "Get TDF - Parameters.vi"("reference in"=w570, "error in (no error)"=w569) -> ("TDF Parameters"=w574:T7, "reference out"=w575:refnum<class "GSwFormDSP.lvclass">, "error out"=w576:errorcluster)  [unwired: 15 in]
            n253 = Bundle By Name(cluster=w574, "Order"=w572) -> (w577:T7)
            n254 = call "Set TDF - Parameters.vi"("reference in"=w575, "error in (no error)"=w576, "TDF Parameters"=w577) -> ("error out"=w573:errorcluster)  [unwired: 14 in, 2 out]
          }
          frame "Fs" {
            # "If there are no signals, we just want to see the design so assume a Fs=44100Hz."
            # "Assume all Fs are = for the design part, if NOT use the lowest one."
            n255 = call "Get - SigMath Data.vi"("reference in"=w596, "error in (no error)"=w595) -> ("SigMath Data"=w597:T6, "error out"=w593:errorcluster)  [unwired: 15 in, 1 out]
            n256 = Unbundle By Name(w597) -> ("GSwFormDSP"=w594:refnum<class "GSwFormDSP.lvclass">)
            n257 = call-dynamic "Get - Fs.vi"("reference in"=w594, "error in (no error)"=w593) -> ("Signals Fs"=w600:dbl[], "error out"=w598:errorcluster)  [unwired: 14 in, 2 out]
            n258 = Array Max & Min(array=w600) -> (min value=w602:dbl)  [unwired: 3 out]
            n259 = Empty Array?(array=w600) -> (empty?=w601:bool)
            n260 = Select(t=44100.0, s=w601, f=w602) -> (s? t:f=→"Fs":dbl)
          }
          frame "Filter Source" {
            n261 = local write "Filter Source"(T1."Custom Filter ..." ("Filter Source")) -> ()
          }
        }
      }
      frame "FP" {
        n262 = case shown="\"Update Graph\"" w606 {
          selector: w606 -> [w611 _ _ _]
          tunnel: w609 -> [_ w619 _ w635]
          tunnel: w608 -> [w612 w618 w629 w636]
          tunnel: [w612 w615 w632 w637] -> w607
          frame "unknown", Default {
            n263 = Concatenate Strings("The following FP Command name is unrecognized:\n", w611) -> (w613:string)
            n264 = One Button Dialog(message=w613) -> ()  [unwired: 1 in, 1 out]
          }
          frame "Open" {
            n265 = call-dynamic "Get VI Ref.vi"("reference in"=w619, "error in (no error)"=w618) -> ("GUI VI Ref"=w616:refnum<vi>, "error out"=w617:errorcluster)  [unwired: 14 in, 2 out]
            n266 = property class="VI"(reference=w616, error in=w617) -> (reference out=w621:refnum<vi>, error out=w622:errorcluster, "Front Panel.Open"=w620:bool)
            n267 = case shown="False" w620 {
              tunnel: [w625 w628] -> w615
              tunnel: w622 -> [w624 w628]
              tunnel: w621 -> [w623 _]
              frame False {
                n268 = invoke class="VI" method="FP.Open"(reference=w623, error in=w624, "Activate"=TRUE, "State"=T4."Standard") -> (error out=w625:errorcluster)  [unwired: 1 in, 4 out]
              }
              frame True {
              }
            }
          }
          frame "Activate Filter Type" {
            n269 = case shown="\"Lowpass\", \"Highpass\", Default" "Filter" {
              tunnel: [T5."Disabled and Grayed Out" ("Disabled") T5."Enabled" ("Disabled")] -> w630
              frame "Lowpass", "Highpass", Default {
              }
              frame "Bandpass", "Bandstop" {
              }
            }
            n270 = property on="Upper Cut Off Freq" class="DigNum (strict)"(error in=w629, "DisabledEnum"=w630) -> (error out=w632:errorcluster)  [unwired: 1 in, 1 out]
          }
          frame "Update Graph" {
            n271 = local read "Fs"() -> (w639:dbl)
            n272 = local read "Filter Source"() -> (w638:T1)
            n273 = case shown="\"Custom Filter ...\", Default" w638 {
              tunnel: [w663 w698] -> w650
              tunnel: w639 -> [w659 w710]
              tunnel: [w651 w699] -> w637
              tunnel: w636 -> [w651 w706]
              tunnel: w635 -> [_ w707]
              frame "Custom Filter ...", Default {
                n274 = local read "Filter"() -> (w658:T3)
                n275 = case shown="\"Elliptic\", Default" "Type" {
                  tunnel: w659 -> [w669 w676 w683 w691 w697]
                  tunnel: "Cut Off Freq" -> [w668 w675 w682 w686 w696]
                  tunnel: "passband ripple (dB)" -> [_ w674 _ w690 _]
                  tunnel: "Order" -> [w667 w673 w680 w689 w695]
                  tunnel: "stopband attenuation (dB)" -> [_ _ w681 w688 _]
                  tunnel: [w666 w672 w679 w687 w694] -> w661
                  tunnel: w658 -> [w665 w671 w678 w685 w693]
                  tunnel: "Upper Cut Off Freq" -> [w664 w670 w677 w684 w692]
                  frame "Butterworth" {
                    n276 = call <vilib>:"Butterworth Coefficients.vi"("order"=w667, "filter type"=w665, "low cutoff freq: fl"=w668, "high cutoff freq: fh"=w664, "sampling freq: fs"=w669) -> ("IIR Filter Cluster"=w666:T8)  [unwired: 5 in, 1 out]
                  }
                  frame "Chebyshev" {
                    n277 = call <vilib>:"Chebyshev Coefficients.vi"("order"=w673, "filter type"=w671, "ripple(dB)"=w674, "low cutoff freq: fl"=w675, "high cutoff freq: fh"=w670, "sampling freq: fs"=w676) -> ("IIR Filter Cluster"=w672:T8)  [unwired: 4 in, 1 out]
                  }
                  frame "Inv Chebyshev" {
                    n278 = call <vilib>:"Inv Chebyshev Coefficients.vi"("order"=w680, "filter type"=w678, "attenuation (dB)"=w681, "low cutoff freq: fl"=w682, "high cutoff freq: fh"=w677, "sampling freq: fs"=w683) -> ("IIR Filter Cluster"=w679:T8)  [unwired: 4 in, 1 out]
                  }
                  frame "Elliptic", Default {
                    n279 = call <vilib>:"Elliptic Coefficients.vi"("stopband attenuation (dB)"=w688, "order"=w689, "filter type"=w685, "passband ripple (dB)"=w690, "low cutoff freq: fl"=w686, "high cutoff freq: fh"=w684, "sampling freq: fs"=w691) -> ("IIR Filter Cluster"=w687:T8)  [unwired: 3 in, 1 out]
                  }
                  frame "Bessel" {
                    n280 = call <vilib>:"Bessel Coefficients.vi"("order"=w695, "filter type"=w693, "low cutoff freq: fl"=w696, "high cutoff freq: fh"=w692, "sampling freq: fs"=w697) -> ("IIR Filter Cluster"=w694:T8)  [unwired: 5 in, 1 out]
                  }
                }
                n281 = To Long Integer(number=w659) -> (32bit integer=w660:i32)
                n282 = call <vilib>:"Impulse Pattern.vi"("samples"=w660) -> ("Impulse Pattern"=w662:dbl[])  [unwired: 2 in, 1 out]
                n283 = call-poly <vilib>:"IIR Cascade Filter.vi"("IIR Filter Cluster"=w661, "X"=w662) -> ("Filtered X"=w663:dbl[])  [unwired: 1 in, 1 out]
              }
              frame "Import Impulse Response (TDMS File)" {
                n284 = call "Get - SigMath Data.vi"("reference in"=w707, "error in (no error)"=w706) -> ("SigMath Data"=w708:T6, "error out"=w700:errorcluster)  [unwired: 15 in, 1 out]
                n285 = Unbundle By Name(w708) -> ("GSwFormDSP"=w705:refnum<class "GSwFormDSP.lvclass">)
                n286 = To Long Integer(number=w710) -> (32bit integer=w709:i32)
                n287 = call <vilib>:"Impulse Pattern.vi"("samples"=w709) -> ("Impulse Pattern"=w704:dbl[])  [unwired: 2 in, 1 out]
                n288 = call "Get TDF - Filter Impulse Response.vi"("reference in"=w705, "error in (no error)"=w700) -> ("Filter Impulse Response (TDF)"=w701:waveform(dbl), "error out"=w699:errorcluster)  [unwired: 15 in, 1 out]
                n289 = Unbundle By Name(w701) -> ("Y"=w702:dbl[])
                n290 = call-poly <vilib>:"Convolution.vi"("algorithm"=enum32{"direct", "frequency domain"}."direct", "Y"=w704, "X"=w702) -> ("X * Y"=w698:dbl[])  [unwired: 7 in, 1 out]
              }
            }
            n291 = Divide(x=w639, y=2.0) -> (x/y=w646:dbl)
            n292 = To Double Precision Complex(1:w650) -> (0:w644:cdb[])
            n293 = Increment(x=w646) -> (x+1=w647:dbl)
            n294 = call-poly <vilib>:"FFT.vi"("X"=w644) -> ("FFT {X}"=w645:cdb[])  [unwired: 2 in, 8 out]
            n295 = To Long Integer(number=w647) -> (32bit integer=w648:i32)
            n296 = Array Subset(array=w645, length=w648) -> (w649:cdb[])  [unwired: 1 in]
            n297 = Complex To Polar(r * e^(i*theta)=w649) -> (r=→"Magnitude Graph":dbl[], theta=w642:dbl[])
            n298 = call <vilib>:"Unwrap Phase.vi"("Phase"=w642) -> ("Unwrapped Phase"=→"Phase Graph":dbl[])  [unwired: 1 in, 9 out]
          }
        }
      }
      frame "---- GUI Functions ----" {
      }
      frame "GUI: Initialize Ref" {
        n299 = control-ref of="GUI Reference"() -> (w715:refnum<vi>)
        n300 = call "Set VI Ref.vi"("reference in"=w720, "error in (no error)"=w716, "GUI VI Ref"=w715) -> ("reference out"=w719:refnum<class "SigMath.lvclass">, "error out"=w714:errorcluster)  [unwired: 15 in]
        n301 = call "Set Close Panel (Yes or No).vi"("reference in"=w719, "error in (no error)"=w714) -> ("reference out"=w718:refnum<class "SigMath.lvclass">, "error out"=w713:errorcluster)  [unwired: 16 in]
        n302 = call "Set Message Window Ref.vi"("reference in"=w718, "error in (no error)"=w713) -> ("error out"=w717:errorcluster)  [unwired: 16 in, 1 out]
      }
      frame "GUI: Exit" {
        n303 = call-dynamic "Get Message Window Ref.vi"("reference in"=w733, "error in (no error)"=w730) -> ("reference out"=w732:refnum<class "SigMath.lvclass">, "Msg Win Ref"=w728:refnum<vi>, "error out"=w731:errorcluster)  [unwired: 15 in]
        n304 = call-dynamic "Get VI Ref.vi"("reference in"=w732, "error in (no error)"=w731) -> ("reference out"=w736:refnum<class "SigMath.lvclass">, "GUI VI Ref"=w734:refnum<vi>, "error out"=w735:errorcluster)  [unwired: 14 in, 1 out]
        n305 = call-dynamic "Get Close Panel (Yes or No).vi"("reference in"=w736, "error in (no error)"=w735) -> ("Close Panel?"=w737:bool, "reference out"=w726:refnum<class "SigMath.lvclass">, "error out"=w727:errorcluster)  [unwired: 15 in]
        n306 = call-dynamic "Get OBJ NOT RefNum.vi"("reference in"=w726, "error in (no error)"=w727) -> ("OBJ not a refnum?"=w723:bool, "reference out"=w725:refnum<class "SigMath.lvclass">, "error out"=w724:errorcluster)  [unwired: 15 in]
        n307 = case shown="True" w723 {
          tunnel: [w742 w745] -> w722
          tunnel: w725 -> [_ w744]
          tunnel: w724 -> [w742 w743]
          frame False {
            # "The OBJ already exist, indicating this is a dialog box or sub-vi so do NOT destroy the original OBJ."
          }
          frame True {
            # "New OBJ was created, so it needs to be deleted."
            n308 = call-dynamic "Destroy.vi"("reference in"=w744, "error in (no error)"=w743) -> ("error out"=w746:errorcluster)  [unwired: 16 in, 1 out]
            n309 = disable-structure shown="Disabled" {
              disable-tunnel: w746 -> [w748 w749]
              disable-tunnel: [w747 w749] -> w745
              frame Disabled {
                # "Enable when NEEDED"
                n310 = call <vilib>:"GarbageCollector.vi"("error in (no error)"=w748) -> ("error out"=w747:errorcluster)  [unwired: 16 in, 2 out]
              }
              frame Enabled {
              }
            }
          }
        }
        n311 = Close Reference(reference=w728, error in (no error)=w722) -> (error out=w740:errorcluster)
        n312 = case shown="True" w737 {
          tunnel: w740 -> [w751 w755]
          tunnel: [w751 w754] -> w738
          tunnel: [w750 w753] -> w739
          tunnel: w734 -> [w750 w752]
          frame False {
          }
          frame True {
            n313 = property class="VI"(reference=w752, error in=w755) -> (reference out=w757:refnum<vi>, error out=w756:errorcluster, "Front Panel.Open"=w758:bool)
            n314 = case shown="True" w758 {
              tunnel: [w760 w764] -> w754
              tunnel: w756 -> [w760 w763]
              tunnel: w757 -> [w759 w762]
              tunnel: [w759 w761] -> w753
              frame False {
              }
              frame True {
                n315 = invoke class="VI" method="FP.Close"(reference=w762, error in=w763) -> (reference out=w761:refnum<vi>, error out=w764:errorcluster)  [unwired: 1 in, 1 out]
              }
            }
          }
        }
        n316 = Close Reference(reference=w739, error in (no error)=w738) -> (error out=w729:errorcluster)
      }
      frame "SEND MSG" {
        n317 = call-dynamic "Get Message Window Ref.vi"("reference in"=w769, "error in (no error)"=w768) -> ("Msg Win Ref"=w765:refnum<vi>, "error out"=w767:errorcluster)  [unwired: 15 in, 1 out]
        n318 = property class="VI"(reference=w765, error in=w767) -> (reference out=w771:refnum<vi>, error out=w770:errorcluster, "Front Panel.Open"=w772:bool)
        n319 = case shown="False" w772 {
          tunnel: [w786 w790] -> w774
          tunnel: w770 -> [w781 w790]
          tunnel: w771 -> [w783 w789]
          tunnel: [w785 w789] -> w773
          frame False {
            w784 = FALSE ("Wait Until Done")
            n320 = invoke class="VI" method="Run VI"(reference=w783, error in=w781, "Wait until done"=w784, "Auto Dispose Ref"=w784) -> (reference out=w782:refnum<vi>, error out=w780:errorcluster)  [unwired: 1 in, 3 out]
            n321 = invoke class="VI" method="FP.Open"(reference=w782, error in=w780, "Activate"=TRUE, "State"=T4."Standard") -> (reference out=w785:refnum<vi>, error out=w786:errorcluster)  [unwired: 1 in, 3 out]
          }
          frame True {
          }
        }
        n322 = Concatenate Strings("\r\n", w778) -> (w777:string)
        n323 = invoke class="VI" method="Ctrl Val.Set"(reference=w773, error in=w774, "Control Name"="Message", "Value"=w777) -> (error out=w766:errorcluster)  [unwired: 1 in, 4 out]
      }
      frame "CLOSE MSG" {
        n324 = call-dynamic "Get Message Window Ref.vi"("reference in"=w794, "error in (no error)"=w795) -> ("Msg Win Ref"=w792:refnum<vi>, "error out"=w793:errorcluster)  [unwired: 15 in, 1 out]
        n325 = property class="VI"(reference=w792, error in=w793) -> (reference out=w799:refnum<vi>, error out=w800:errorcluster, "Front Panel.Open"=w798:bool)
        n326 = case shown="True" w798 {
          tunnel: [w803 w807] -> w797
          tunnel: w800 -> [w803 w806]
          tunnel: w799 -> [w802 w805]
          tunnel: [w802 w804] -> w796
          frame False {
          }
          frame True {
            n327 = invoke class="VI" method="FP.Close"(reference=w805, error in=w806) -> (reference out=w804:refnum<vi>, error out=w807:errorcluster)  [unwired: 1 in, 1 out]
          }
        }
        n328 = invoke class="VI" method="Abort VI"(reference=w796, error in=w797) -> (error out=w791:errorcluster)  [unwired: 1 in, 2 out]
      }
      frame "---- Miscelleneous ----" {
      }
      frame "unknown", Default {
        n329 = Concatenate Strings("The following state is unrecognized?\n", w812) -> (w811:string)
        n330 = One Button Dialog(message=w811) -> ()  [unwired: 1 in, 1 out]
      }
      frame "Error" {
        n331 = call <vilib>:"General Error Handler.vi"("error in (no error)"=w815) -> ()  [unwired: 10 in, 5 out]
      }
      frame "Next" {
        # "This is an empty case used so the queue does NOT stop if there is an empty string between two valid states!"
      }
      frame "Quit" {
        # "WARNING!, If the state machine crash, then it will also \"Quit\"??"
        # "This is the case used to simply exit when this GUI is used as a SubVI!"
        n332 = call-dynamic "Destroy.vi"("reference in"=w822, "error in (no error)"=w821) -> ("error out"=w820:errorcluster)  [unwired: 16 in, 1 out]
      }
    }
    "State Index" <- w17
  }
  "error out" <- w2
